vi "Update Exp Cluster by ref.vi"(8 "Error In":errorcluster, 10 "Exp 1":T1, 11 "Controls[]":refnum<vi>[](array[refnum])) -> (0 "Error Out":errorcluster)   [LabVIEW 2013]
uses:
  Controls/Individual User Inputs_MultiTest.ctl
  Controls/Test Selection.ctl
panel:
  # "Calculation Settings"
  # "Test Settings"
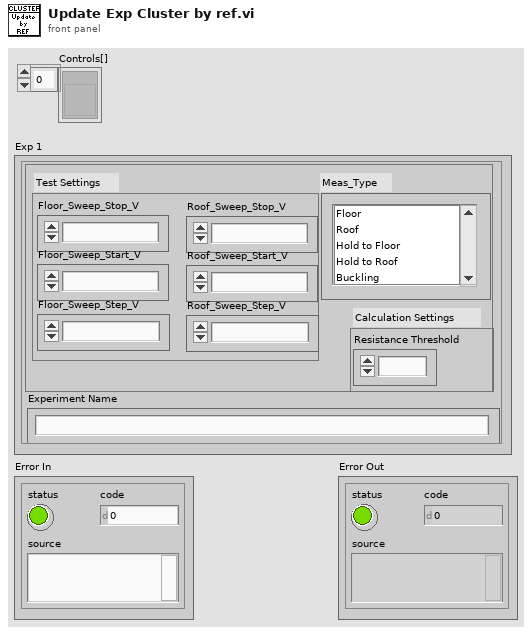
[diagram p1: front panel]
types:
  T1 = typedef "Individual User Inputs_MultiTest.ctl" = cluster{"Floor_Sweep_Stop_V":dbl, "Resistance Threshold":dbl, "Floor_Sweep_Start_V":dbl, "Floor_Sweep_Step_V":dbl, "Roof_Sweep_Stop_V":dbl, "Roof_Sweep_Start_V":dbl, "Roof_Sweep_Step_V":dbl, "Experiment Name":string, "Meas_Type":T2}
  T2 = typedef "Test Selection.ctl" = i32[]
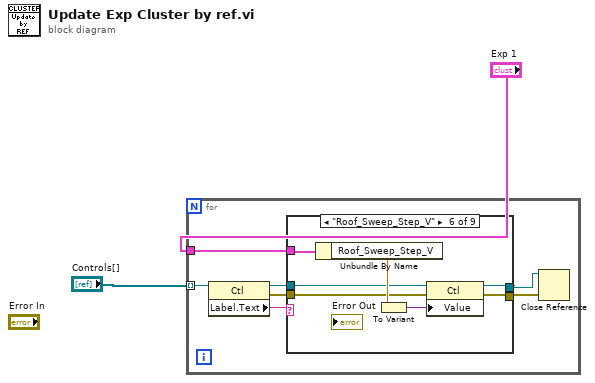
[diagram p0: block diagram]
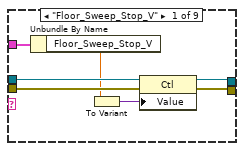
[diagram p2: hidden frame]
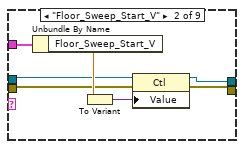
[diagram p3: hidden frame]
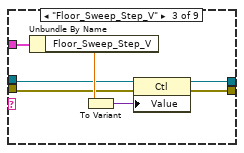
[diagram p4: hidden frame]
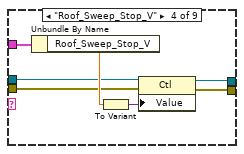
[diagram p5: hidden frame]
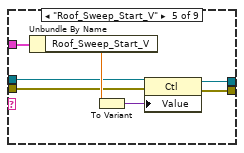
[diagram p6: hidden frame]
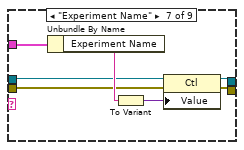
[diagram p7: hidden frame]
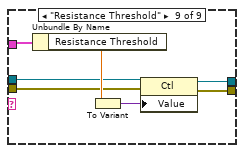
[diagram p9: hidden frame]
diagram:
  n1 = for {
    tunnel: "Controls[]" -> [w9] mode=indexing
    tunnel: "Exp 1" -> [w5]
    n2 = property class="Ctl"(reference=w9) -> (reference out=w7:refnum<vi>, error out=w6:errorcluster, "Label.Text"=w8:string)  [unwired: 1 in]
    n3 = case shown="\"Roof_Sweep_Step_V\"" w8 {
      tunnel: w7 -> [w16 w19 w26 w35 w41 w48 w55 w60 w64]
      tunnel: w6 -> [w15 w20 w27 w34 w42 w47 w54 w59 w65]
      tunnel: w5 -> [w14 w21 w28 w33 w40 w49 w56 _ w63]
      tunnel: [w11 w17 w24 w31 w38 w45 w53 w59 w62] -> w4
      tunnel: [w10 w18 w25 w32 w39 w46 w52 w60 w61] -> w3
      frame "Floor_Sweep_Stop_V" {
        n4 = Unbundle By Name(w14) -> ("Floor_Sweep_Stop_V"=w13:dbl)
        n5 = To Variant(anything=w13) -> (Variant=w12:variant)
        n6 = property class="Ctl"(reference=w16, error in=w15, "Value"=w12) -> (reference out=w10:refnum<vi>, error out=w11:errorcluster)
      }
      frame "Floor_Sweep_Start_V" {
        n7 = Unbundle By Name(w21) -> ("Floor_Sweep_Start_V"=w23:dbl)
        n8 = To Variant(anything=w23) -> (Variant=w22:variant)
        n9 = property class="Ctl"(reference=w19, error in=w20, "Value"=w22) -> (reference out=w18:refnum<vi>, error out=w17:errorcluster)
      }
      frame "Floor_Sweep_Step_V" {
        n10 = Unbundle By Name(w28) -> ("Floor_Sweep_Step_V"=w30:dbl)
        n11 = To Variant(anything=w30) -> (Variant=w29:variant)
        n12 = property class="Ctl"(reference=w26, error in=w27, "Value"=w29) -> (reference out=w25:refnum<vi>, error out=w24:errorcluster)
      }
      frame "Roof_Sweep_Stop_V" {
        n13 = Unbundle By Name(w33) -> ("Roof_Sweep_Stop_V"=w37:dbl)
        n14 = To Variant(anything=w37) -> (Variant=w36:variant)
        n15 = property class="Ctl"(reference=w35, error in=w34, "Value"=w36) -> (reference out=w32:refnum<vi>, error out=w31:errorcluster)
      }
      frame "Roof_Sweep_Start_V" {
        n16 = Unbundle By Name(w40) -> ("Roof_Sweep_Start_V"=w44:dbl)
        n17 = To Variant(anything=w44) -> (Variant=w43:variant)
        n18 = property class="Ctl"(reference=w41, error in=w42, "Value"=w43) -> (reference out=w39:refnum<vi>, error out=w38:errorcluster)
      }
      frame "Roof_Sweep_Step_V" {
        n19 = Unbundle By Name(w49) -> ("Roof_Sweep_Step_V"=w51:dbl)
        n20 = To Variant(anything=w51) -> (Variant=w50:variant)
        n21 = property class="Ctl"(reference=w48, error in=w47, "Value"=w50) -> (reference out=w46:refnum<vi>, error out=w45:errorcluster)
      }
      frame "Experiment Name" {
        n22 = Unbundle By Name(w56) -> ("Experiment Name"=w58:string)
        n23 = To Variant(anything=w58) -> (Variant=w57:variant)
        n24 = property class="Ctl"(reference=w55, error in=w54, "Value"=w57) -> (reference out=w52:refnum<vi>, error out=w53:errorcluster)
      }
      frame "Meas_Type", Default {
      }
      frame "Resistance Threshold" {
        n25 = Unbundle By Name(w63) -> ("Resistance Threshold"=w67:dbl)
        n26 = To Variant(anything=w67) -> (Variant=w66:variant)
        n27 = property class="Ctl"(reference=w64, error in=w65, "Value"=w66) -> (reference out=w61:refnum<vi>, error out=w62:errorcluster)
      }
    }
    n28 = Close Reference(reference=w3, error in (no error)=w4) -> ()  [unwired: 1 out]
  }
